vi "MessageProcessingDraft.vi"() -> ()   [LabVIEW 2011]
uses:
  Typedefs/missionResults.ctl
panel:
  out "Mission Results":T1[](array[typedef])
  out "Total time (s)":dbl
  out "Run end":timestamp
  out "Run start":timestamp
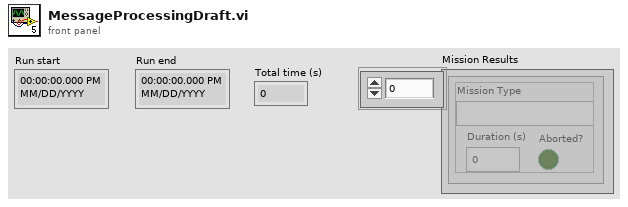
[diagram p1: front panel]
types:
  T1 = typedef "missionResults.ctl" = cluster{"Mission Type":string, "Duration (s)":dbl, "Aborted?":bool}
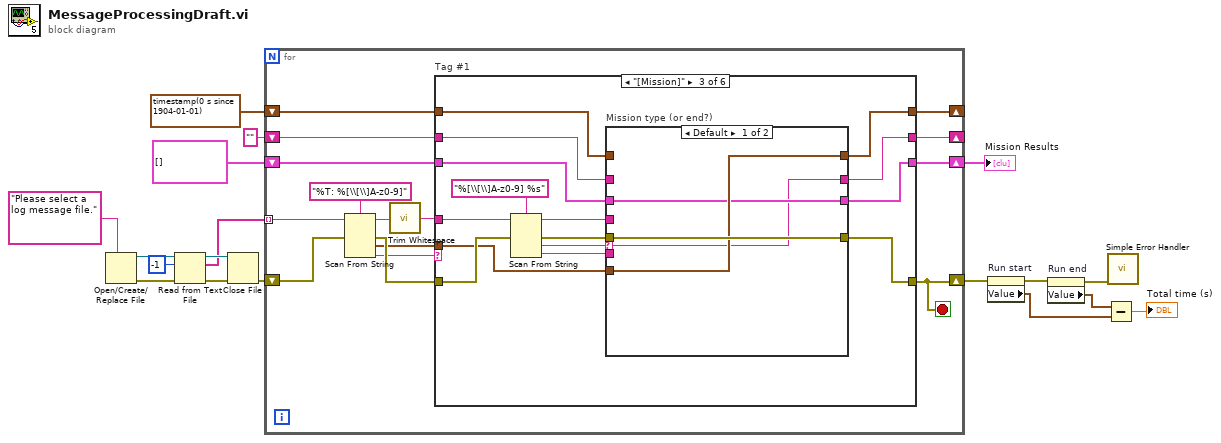
[diagram p0: block diagram]
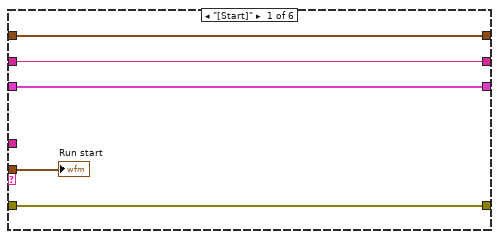
[diagram p2: hidden frame]
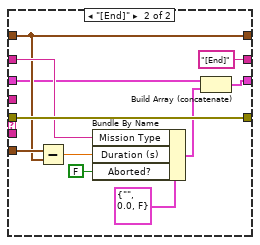
[diagram p4: hidden frame]
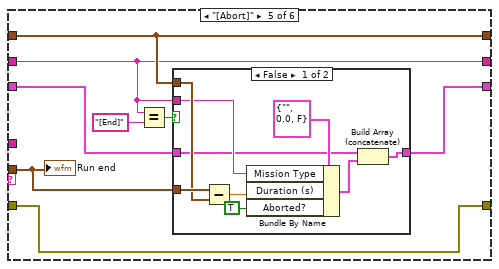
[diagram p6: hidden frame]
diagram:
  n1 = Open/Create/Replace File(prompt="Please select a log message file.") -> (refnum out=w17:refnum<file>, error out=w16:errorcluster)  [unwired: 5 in, 1 out]
  n2 = Read from Text File(file (use dialog)=w17, count=-1, error in=w16) -> (refnum out=w14:refnum<file>, text=w12:string[], error out=w13:errorcluster)  [unwired: 1 in, 1 out]
  n3 = Close File(refnum=w14, error in=w13) -> (error out=w11:errorcluster)  [unwired: 1 out]
  n4 = for {
    tunnel: w12 -> [w33] mode=indexing
    shift-right: [w28] -> w10
    shift-left: w11 -> [w32]
    shift-right: [w20] -> w1
    shift-left: T1[] [] ("Mission Results") -> [w24]
    shift-right: [w22] -> _
    shift-left: timestamp(0 s since 1904-01-01) ("output 1") -> [w23]
    shift-right: [w19] -> _
    shift-left: "" ("remaining string") -> [w21]
    stop <- w28 stop-if-true
    n5 = Scan From String(format string="%T: %[\\[\\]A-z0-9]", input string=w33, error in=w32) -> (remaining string=w26:string, error out=w30:errorcluster, output 1=w29:timestamp, output 2=w27:string)  [unwired: 3 in, 1 out]
    n6 = call <vilib>:"Trim Whitespace.vi"("string"=w26) -> ("trimmed string"=w25:string)  [unwired: 1 in]
    n7 = case "Tag #1" shown="\"[Mission]\"" w27 {
      tunnel: w30 -> [w37 w42 w55 w76 w79 w98]
      tunnel: [w37 w42 w52 w76 w79 w98] -> w28
      tunnel: w29 -> [w38 _ w49 _ w80 _]
      tunnel: w25 -> [_ _ w57 _ _ _]
      tunnel: w24 -> [w34 w39 w46 w73 w82 w95]
      tunnel: w23 -> [w36 w41 w48 w75 w78 w97]
      tunnel: [w36 w41 w47 w75 w78 w97] -> w22
      tunnel: w21 -> [w35 w40 w45 w74 w77 w96]
      tunnel: [w34 w39 w44 w73 w81 w95] -> w20
      tunnel: [w35 w40 w43 w74 w77 w96] -> w19
      frame "[Start]" {
        "Run start" <- w38
      }
      frame "[User]" {
      }
      frame "[Mission]" {
        n8 = Scan From String(format string="%[\\[\\]A-z0-9] %s", input string=w57, error in=w55) -> (remaining string=w50:string, error out=w53:errorcluster, output 1=w54:string, output 2=w51:string)  [unwired: 3 in, 1 out]
        n9 = case "Mission type (or end?)" shown="Default" w54 {
          selector: w54 -> [w58 _]
          tunnel: w53 -> [w61 w71]
          tunnel: [w61 w71] -> w52
          tunnel: w51 -> [_ _]
          tunnel: w50 -> [_ _]
          tunnel: w49 -> [w60 w68]
          tunnel: w48 -> [_ w67]
          tunnel: [w60 w67] -> w47
          tunnel: w46 -> [w59 w65]
          tunnel: w45 -> [_ w70]
          tunnel: [w59 w63] -> w44
          tunnel: [w58 "[End]"] -> w43
          frame Default {
          }
          frame "[End]" {
            n10 = Subtract(x=w68, y=w67) -> (x-y=w66:dbl)
            n11 = Bundle By Name(cluster=T1 {"Mission Type"="", "Duration (s)"=0.0, "Aborted?"=FALSE} ("Cluster"), "Mission Type"=w70, "Duration (s)"=w66, "Aborted?"=FALSE) -> (w64:T1)
            n12 = Build Array (concatenate)(w65, w64) -> (w63:T1[])
          }
        }
      }
      frame "[Waypoint]" {
      }
      frame "[Abort]" {
        n13 = Equal?(x=w77, y="[End]") -> (x = y?=w84:bool)
        n14 = case shown="False" w84 {
          tunnel: w77 -> [w88 _]
          tunnel: w82 -> [w87 w94]
          tunnel: [w85 w94] -> w81
          tunnel: w80 -> [w90 _]
          tunnel: w78 -> [w89 _]
          frame False {
            n15 = Subtract(x=w90, y=w89) -> (x-y=w91:dbl)
            n16 = Bundle By Name(cluster=T1 {"Mission Type"="", "Duration (s)"=0.0, "Aborted?"=FALSE} ("Cluster"), "Mission Type"=w88, "Duration (s)"=w91, "Aborted?"=TRUE) -> (w86:T1)
            n17 = Build Array (concatenate)(w87, w86) -> (w85:T1[])
          }
          frame True {
          }
        }
        "Run end" <- w80
      }
      frame Default {
      }
    }
  }
  "Mission Results" <- w1
  n18 = property on="Run start" class="AbsTime (strict)"(error in=w10) -> (error out=w9:errorcluster, "Value"=w6:timestamp)  [unwired: 1 in, 1 out]
  n19 = property on="Run end" class="AbsTime (strict)"(error in=w9) -> (error out=w8:errorcluster, "Value"=w7:timestamp)  [unwired: 1 in, 1 out]
  n20 = Subtract(x=w7, y=w6) -> (x-y=→"Total time (s)":dbl)
  n21 = call <vilib>:"Simple Error Handler.vi"("error in (no error)"=w8) -> ()  [unwired: 4 in, 5 out]
